vi "Desired Position.vi"(0 "FT":dbl[](array[numeric])=[0.0, 0.0, 0.0], 1 "v10":dbl[](array[numeric])=[-1.0, 0.0, 0.0], 2 "v20":dbl[](array[numeric])=[-1.0, 0.0, 0.0], 3 "v30":dbl[](array[numeric])=[-1.0, 0.0, 0.0], 5 "damping":dbl[](array[numeric])=[0.0, 0.0, 0.0], 7 "radius":dbl=10.0, 9 "dt":dbl=0.001, 11 "R":T1) -> (4 "v1d":dbl[](array[numeric]) format="%.2f", 6 "v2d":dbl[](array[numeric]) format="%.2f", 8 "v3d":dbl[](array[numeric]) format="%.2f", 10 "R'":T1)   [LabVIEW 2017]
uses:
  <vilib>/Analysis/Matrix/Datatypes/RealMatrix.ctl
  <vilib>/Analysis/baseanly.llb/Real A x B.vi
  <vilib>/Analysis/baseanly.llb/A x Vector.vi
  <vilib>/Analysis/_algsub.llb/Vector Norm.vi
  <vilib>/Analysis/_algsub.llb/Real Vector Norm.vi
  <vilib>/Analysis/baseanly.llb/Outer Product.vi
  <vilib>/Analysis/baseanly.llb/Real Outer Product.vi
  <vilib>/robotics/Kinematics/Create Lie Group Matrix.vi
  <vilib>/Analysis/7linalg.llb/Create Special Matrix.vi
  <vilib>/Analysis/7linalg.llb/Create Special Real Matrix.vi
  <vilib>/Analysis/Matrix/Numeric/Multiply/Multiply.vi
  <vilib>/Analysis/Matrix/Numeric/Multiply/Multiply - RM,R.vi
  <vilib>/Analysis/Matrix/Numeric/Multiply/Multiply - R,RM.vi
  <vilib>/Analysis/Matrix/Numeric/Add/Add.vi
  <vilib>/Analysis/Matrix/Numeric/Add/Add - RM,RM.vi
  <vilib>/robotics/Kinematics/NI_Kinematics.lvlib
  <vilib>/Analysis/NI_AALBase.lvlib
  <vilib>/Analysis/Matrix/NI_Matrix.lvlib
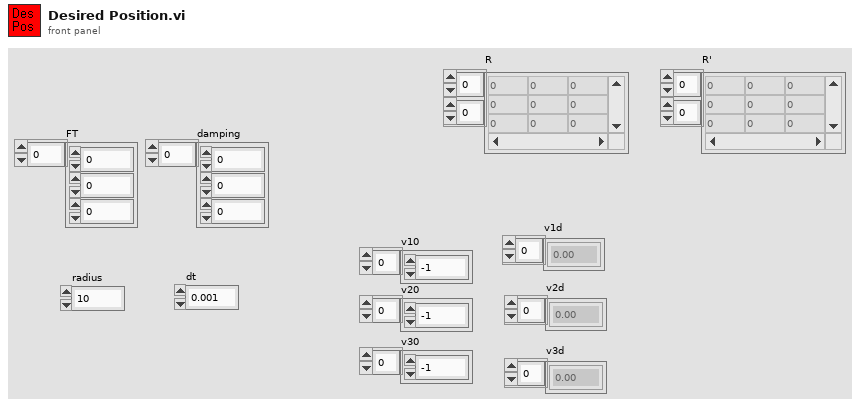
[diagram p1: front panel]
types:
  T1 = typedef "NI_Matrix.lvlib/RealMatrix.ctl" = dbl[][]
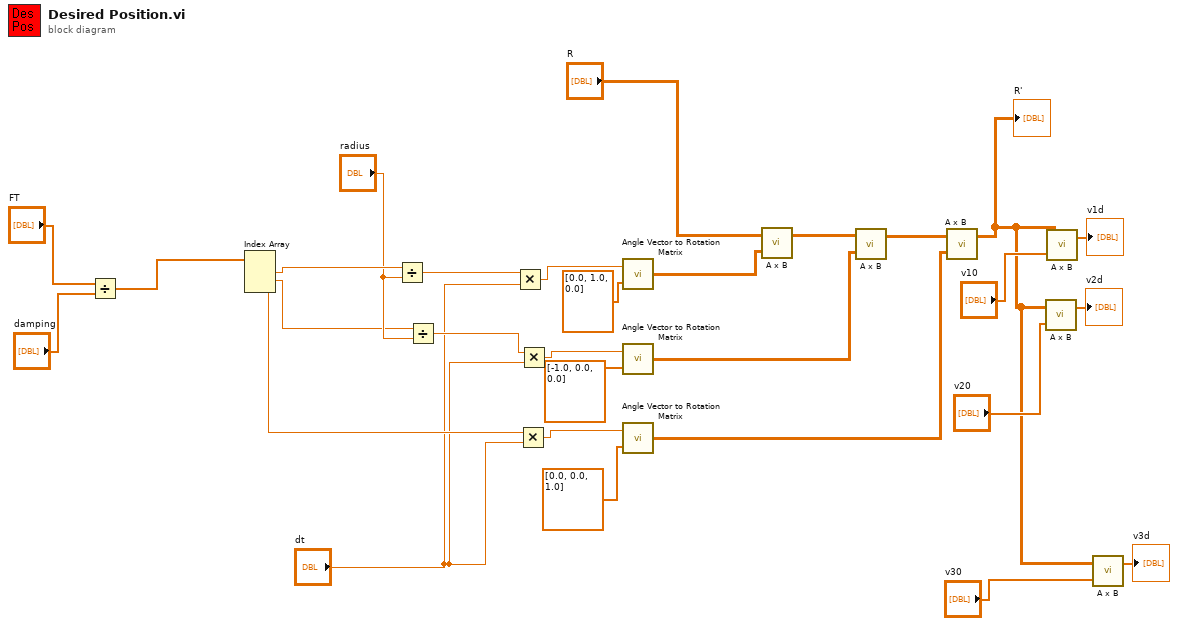
[diagram p0: block diagram]
diagram:
  n1 = Divide(x="FT", y="damping") -> (x/y=w27:dbl[])
  n2 = Index Array(array=w27) -> (element #1=w26:dbl, element #2=w24:dbl, element #3=w21:dbl)  [unwired: 3 in]
  n3 = Divide(x=w26, y="radius") -> (x/y=w23:dbl)
  n4 = Divide(x=w24, y="radius") -> (x/y=w22:dbl)
  n5 = Multiply(x=w23, y="dt") -> (x*y=w19:dbl)
  n6 = Multiply(x=w21, y="dt") -> (x*y=w17:dbl)
  n7 = Multiply(x=w22, y="dt") -> (x*y=w18:dbl)
  n8 = call <vilib>:"Angle Vector to Rotation Matrix.vi"("vector"=dbl[] [0.0, 1.0, 0.0], "angle"=w19) -> ("rotation matrix"=w12:T1)
  n9 = call <vilib>:"Angle Vector to Rotation Matrix.vi"("vector"=dbl[] [-1.0, 0.0, 0.0], "angle"=w18) -> ("rotation matrix"=w10:T1)
  n10 = call <vilib>:"Angle Vector to Rotation Matrix.vi"("vector"=dbl[] [0.0, 0.0, 1.0], "angle"=w17) -> ("rotation matrix"=w8:T1)
  n11 = call-poly <vilib>:"A x B.vi"("B"=w12, "A"="R") -> ("A x B"=w11:T1)  [unwired: 1 out]
  n12 = call-poly <vilib>:"A x B.vi"("B"=w10, "A"=w11) -> ("A x B"=w9:T1)  [unwired: 1 out]
  n13 = call-poly <vilib>:"A x B.vi"("B"=w8, "A"=w9) -> ("A x B"=w5:T1)  [unwired: 1 out]
  "R'" <- w5
  n14 = call-poly <vilib>:"A x B.vi"("Vector"="v20", "A"=w5) -> ("A x Vector"=→"v2d":dbl[])  [unwired: 1 out]
  n15 = call-poly <vilib>:"A x B.vi"("Vector"="v10", "A"=w5) -> ("A x Vector"=→"v1d":dbl[])  [unwired: 1 out]
  n16 = call-poly <vilib>:"A x B.vi"("Vector"="v30", "A"=w5) -> ("A x Vector"=→"v3d":dbl[])  [unwired: 1 out]
